vi "SEK2020v1SubVIIrParaOrigem00.vi"(8 "Parâmetros":T1={"Azul Max EV3 Cor"=17, "Azul Min EV3 Cor"=0, "Verde Max EV3 Cor"=6, "Verde Min EV3 Cor"=0, "Vermelho Max Ev3 Cor"=0, "Vermelho Min EV3 Cor"=0, "Chão EV3 Cor"=0.0, "Branco Max EV3 Cor"=0.0, "Branco Min EV3 Cor"=0.0, "Preto Max EV3 Cor"=0.0, "Preto Min EV3 Cor"=0.0, "Distância Tubulação"=0.0, "Distância Frontal"=0.0, "Amarelo Max EV3 Cor"=0.0, "Amarelo Min EV3 Cor"=0.0, "Distância Lateral"=0.0, "90°"=0.0, "180°"=0.0, "Seguidor de Linha"=0.0}, 11 "NXT/EV3":T2) -> (3 "NXT/EV3 2":T2)   [LabVIEW 2016]
uses:
  <vilib>/NXT/Subs/LVHSConnector.ctl
  <vilib>/NXT/LegoClasses/BrickReference/BrickReference.lvclass
  <vilib>/NXT/Block Support/NXT_OutputPort.ctl
  <vilib>/NXT/Block Support/NXT_InputPort.ctl
  <vilib>/NXT/Dual Mode Library/Sensors/EV3_Color_Reflect.vi
  <vilib>/NXT/NXTIO Xnodes/NXTIONodeSubVIs/NXTStopMotors.vi
  <vilib>/NXT/NXTIO Xnodes/AddressXNode/NXTIOAddress.xnode
  <vilib>/NXT/NXTIO Xnodes/NXTIOXNode/NXTIO.xnode
panel:
  out "x+1":i32
  in  "x":i32
  # "Sensor EV3 Cor"
  # "Sensor Ultrassônico"
  # "Sensor Giroscópio"
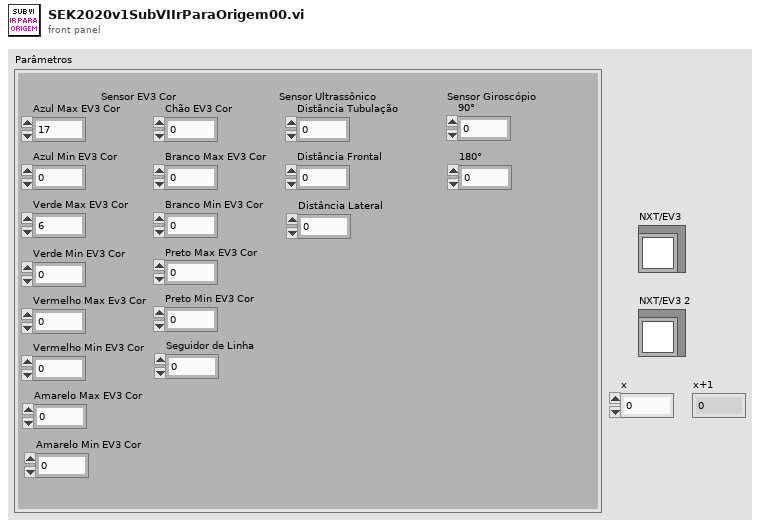
[diagram p1: front panel]
types:
  T1 = cluster{"Azul Max EV3 Cor":i32, "Azul Min EV3 Cor":i32, "Verde Max EV3 Cor":i32, "Verde Min EV3 Cor":i32, "Vermelho Max Ev3 Cor":i32, "Vermelho Min EV3 Cor":i32, "Chão EV3 Cor":sgl, "Branco Max EV3 Cor":sgl, "Branco Min EV3 Cor":sgl, "Preto Max EV3 Cor":sgl, "Preto Min EV3 Cor":sgl, "Distância Tubulação":sgl, "Distância Frontal":sgl, "Amarelo Max EV3 Cor":dbl, "Amarelo Min EV3 Cor":dbl, "Distância Lateral":sgl, "90°":sgl, "180°":sgl, "Seguidor de Linha":dbl}
  T2 = typedef "LVHSConnector.ctl" = refnum<class "BrickReference.lvclass">
  T3 = typedef "NXT_OutputPort.ctl" = u8
  T4 = typedef "NXT_InputPort.ctl" = u32
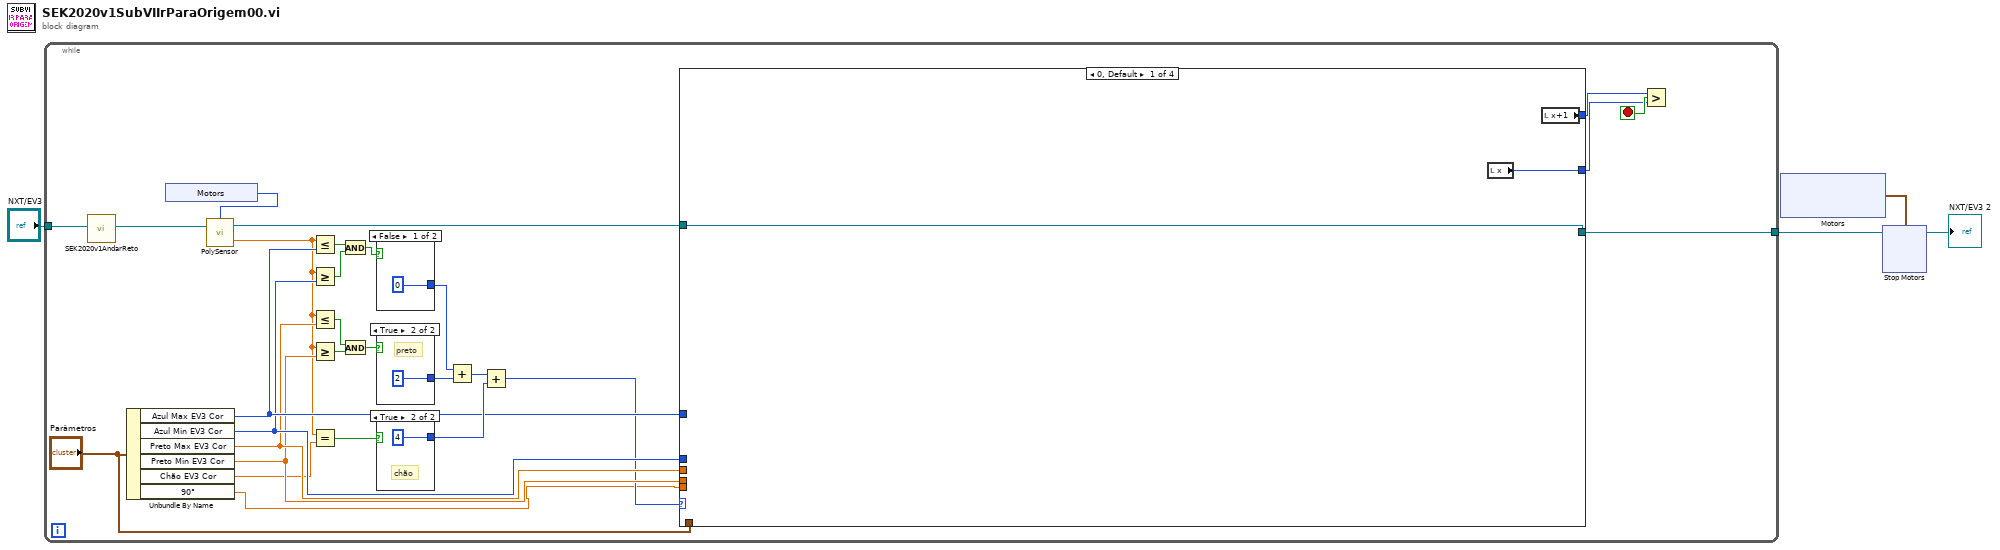
[diagram p0: block diagram]
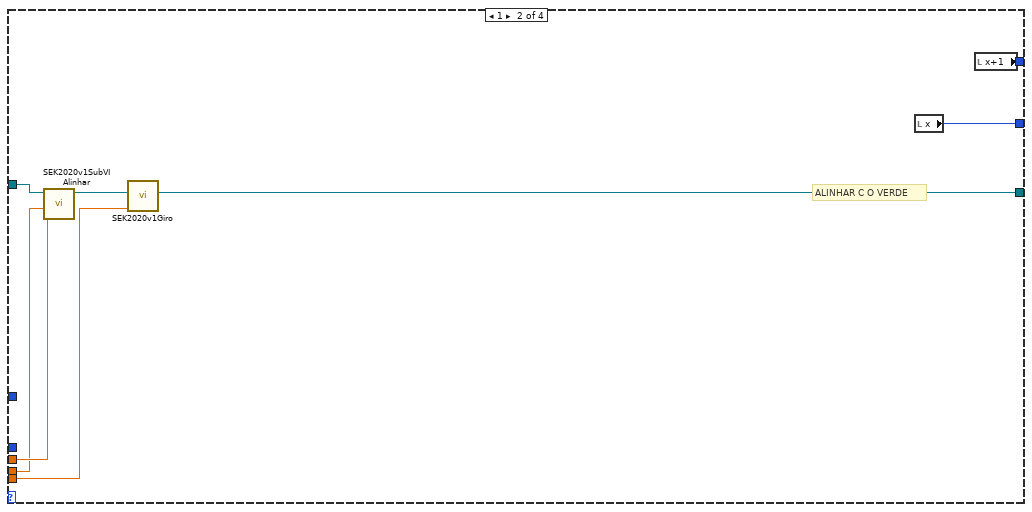
[diagram p2: hidden frame]
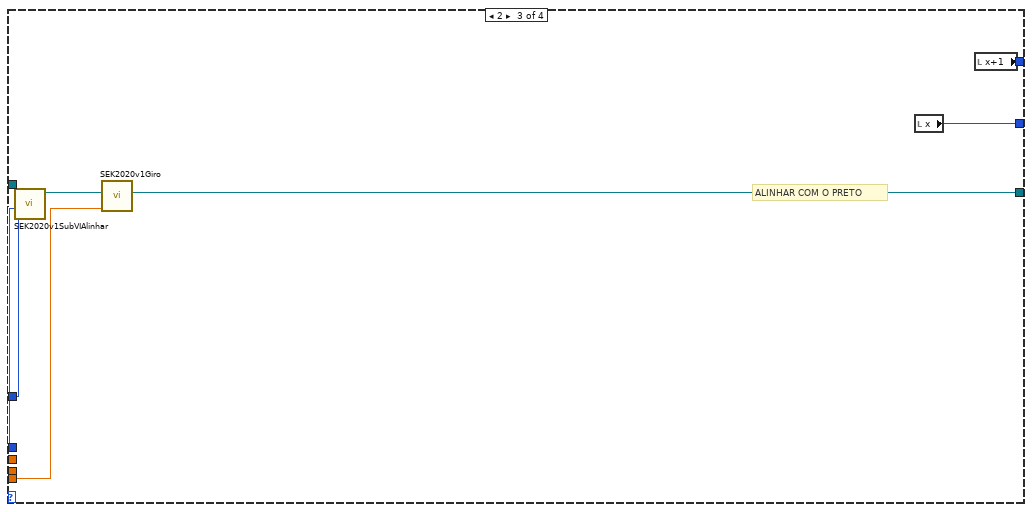
[diagram p3: hidden frame]
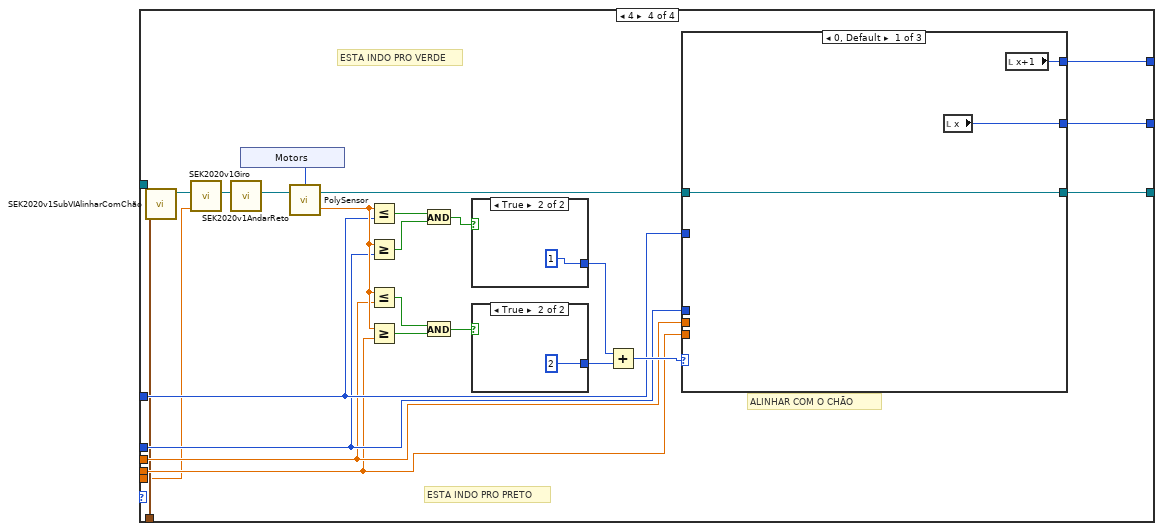
[diagram p4: hidden frame]
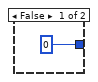
[diagram p5: hidden frame]
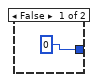
[diagram p6: hidden frame]
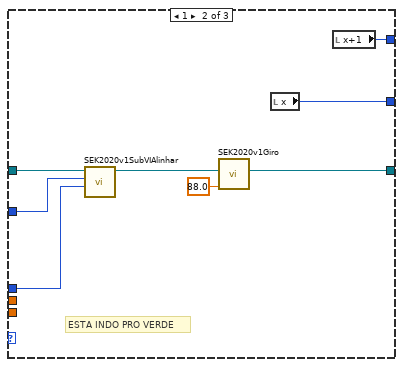
[diagram p7: hidden frame]
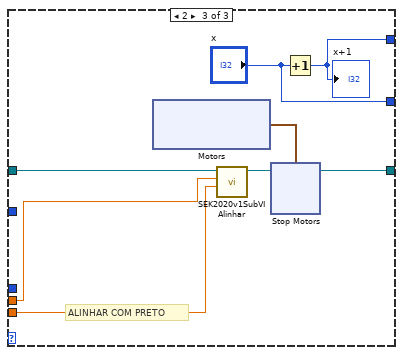
[diagram p8: hidden frame]
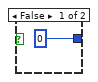
[diagram p9: hidden frame]
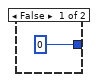
[diagram p10: hidden frame]
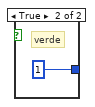
[diagram p11: hidden frame]
diagram:
  n1 = while {
    tunnel: "NXT/EV3" -> [w22]
    tunnel: [w7] -> w1
    stop <- w21 stop-if-true
    n2 = call "SEK2020v1AndarReto.vi"("NXT/EV3"=w22) -> ("NXT/EV3 2"=w10:T2)  [unwired: 9 in]
    n3 = Unbundle By Name("Parâmetros") -> ("Azul Max EV3 Cor"=w20:i32, "Azul Min EV3 Cor"=w19:i32, "Preto Max EV3 Cor"=w18:sgl, "Preto Min EV3 Cor"=w17:sgl, "Chão EV3 Cor"=w15:sgl, "90°"=w6:sgl)
    n4 = xnode "Motors"() -> ("Sensor"=w16:T4)
    n5 = call-poly <vilib>:"PolySensor.vi"("NXT/EV3"=w10, "Port (Port 1)"=w16) -> ("Scaled Value"=w12:sgl, "NXT/EV3"=w8:T2)  [unwired: 1 in]
    n6 = Less Or Equal?(x=w12, y=w20) -> (x <= y?=w25:bool)
    n7 = Greater Or Equal?(x=w12, y=w19) -> (x >= y?=w26:bool)
    n8 = Less Or Equal?(x=w12, y=w18) -> (x <= y?=w28:bool)
    n9 = Greater Or Equal?(x=w12, y=w17) -> (x >= y?=w27:bool)
    n10 = Equal?(x=w12, y=w15) -> (x = y?=w9:bool)
    n11 = And(x=w25, y=w26) -> (x .and. y?=w24:bool)
    n12 = And(x=w28, y=w27) -> (x .and. y?=w23:bool)
    n13 = case shown="False" w24 {
      tunnel: [0 1] -> w32
      frame False {
      }
      frame True {
        # "verde"
      }
    }
    n14 = case shown="True" w23 {
      tunnel: [0 2] -> w31
      frame False {
      }
      frame True {
        # "preto"
      }
    }
    n15 = case shown="True" w9 {
      tunnel: [0 4] -> w30
      frame False {
      }
      frame True {
        # "chão"
      }
    }
    n16 = Add(x=w32, y=w31) -> (x+y=w29:i32)
    n17 = Add(x=w29, y=w30) -> (x+y=w11:i32)
    n18 = case shown="0, Default" w11 {
      tunnel: w20 -> [_ _ w51 w65]
      tunnel: w19 -> [_ _ w52 w64]
      tunnel: w18 -> [_ w44 _ w63]
      tunnel: w17 -> [_ w43 _ w62]
      tunnel: w8 -> [w36 w42 w50 w77]
      tunnel: [w36 w38 w46 w60] -> w7
      tunnel: [w35 w40 w49 w59] -> w14
      tunnel: [w34 w41 w48 w58] -> w13
      tunnel: "Parâmetros" -> [_ _ _ w54]
      tunnel: w6 -> [_ w37 w45 w53]
      frame 0, Default {
        n19 = local read "x"() -> (w35:i32)
        n20 = local read "x+1"() -> (w34:i32)
      }
      frame 1 {
        # "ALINHAR C O VERDE"
        n21 = call "SEK2020v1SubVIAlinhar.vi"("Min EV3 Cor"=w43, "Max EV3 Cor"=w44, "NXT/EV3"=w42) -> ("NXT/EV3 2"=w39:T2)  [unwired: 8 in]
        n22 = call "SEK2020v1Giro.vi"("ANGULO"=w37, "NXT/EV3"=w39) -> ("NXT/EV3 2"=w38:T2)  [unwired: 6 in]
        n23 = local read "x"() -> (w40:i32)
        n24 = local read "x+1"() -> (w41:i32)
      }
      frame 2 {
        # "ALINHAR COM O PRETO"
        n25 = call "SEK2020v1SubVIAlinhar.vi"("Min EV3 Cor"=w52, "Max EV3 Cor"=w51, "NXT/EV3"=w50) -> ("NXT/EV3 2"=w47:T2)  [unwired: 8 in]
        n26 = call "SEK2020v1Giro.vi"("ANGULO"=w45, "NXT/EV3"=w47) -> ("NXT/EV3 2"=w46:T2)  [unwired: 6 in]
        n27 = local read "x"() -> (w49:i32)
        n28 = local read "x+1"() -> (w48:i32)
      }
      frame 4 {
        # "ESTA INDO PRO VERDE"
        # "ESTA INDO PRO PRETO"
        # "ALINHAR COM O CHÃO"
        n29 = call "SEK2020v1SubVIAlinharComChão.vi"("Parâmetros"=w54, "NXT/EV3"=w77) -> ("NXT/EV3 2"=w57:T2)  [unwired: 9 in]
        n30 = call "SEK2020v1Giro.vi"("ANGULO"=w53, "NXT/EV3"=w57) -> ("NXT/EV3 2"=w56:T2)  [unwired: 6 in]
        n31 = call "SEK2020v1AndarReto.vi"("NXT/EV3"=w56) -> ("NXT/EV3 2"=w71:T2)  [unwired: 9 in]
        n32 = xnode "Motors"() -> ("Sensor"=w55:T4)
        n33 = call-poly <vilib>:"PolySensor.vi"("NXT/EV3"=w71, "Port (Port 1)"=w55) -> ("Scaled Value"=w72:sgl, "NXT/EV3"=w61:T2)  [unwired: 1 in]
        n34 = Less Or Equal?(x=w72, y=w65) -> (x <= y?=w73:bool)
        n35 = Greater Or Equal?(x=w72, y=w64) -> (x >= y?=w74:bool)
        n36 = Less Or Equal?(x=w72, y=w63) -> (x <= y?=w76:bool)
        n37 = Greater Or Equal?(x=w72, y=w62) -> (x >= y?=w75:bool)
        n38 = And(x=w73, y=w74) -> (x .and. y?=w70:bool)
        n39 = And(x=w76, y=w75) -> (x .and. y?=w69:bool)
        n40 = case shown="True" w70 {
          tunnel: [0 1] -> w68
          frame False {
          }
          frame True {
          }
        }
        n41 = case shown="True" w69 {
          tunnel: [0 2] -> w67
          frame False {
          }
          frame True {
          }
        }
        n42 = Add(x=w68, y=w67) -> (x+y=w66:i32)
        n43 = case shown="0, Default" w66 {
          tunnel: w65 -> [_ w93 _]
          tunnel: w64 -> [_ w92 _]
          tunnel: w63 -> [_ _ w101]
          tunnel: w62 -> [_ _ w100]
          tunnel: w61 -> [w85 w91 w99]
          tunnel: [w85 w87 w94] -> w60
          tunnel: [w83 w89 w96] -> w58
          tunnel: [w84 w90 "x"] -> w59
          frame 0, Default {
            n44 = local read "x"() -> (w84:i32)
            n45 = local read "x+1"() -> (w83:i32)
          }
          frame 1 {
            # "ESTA INDO PRO VERDE"
            n46 = call "SEK2020v1SubVIAlinhar.vi"("Min EV3 Cor"=w92, "Max EV3 Cor"=w93, "NXT/EV3"=w91) -> ("NXT/EV3 2"=w88:T2)  [unwired: 8 in]
            n47 = call "SEK2020v1Giro.vi"("ANGULO"=sgl 88.0, "NXT/EV3"=w88) -> ("NXT/EV3 2"=w87:T2)  [unwired: 6 in]
            n48 = local read "x"() -> (w90:i32)
            n49 = local read "x+1"() -> (w89:i32)
          }
          frame 2 {
            # "ALINHAR COM PRETO"
            n50 = xnode "Motors"() -> ("Motor"=w98:cluster{"Port":T3, "Port":T3})
            n51 = call "SEK2020v1SubVIAlinhar.vi"("Min EV3 Cor"=w100, "Max EV3 Cor"=w101, "NXT/EV3"=w99) -> ("NXT/EV3 2"=w97:T2)  [unwired: 8 in]
            n52 = xnode "Stop Motors"("Motors"=w98, "NXT/EV3"=w97) -> ("NXT/EV3"=w94:T2)
            n53 = Increment(x="x") -> (x+1=w96:i32)
            "x+1" <- w96
          }
        }
      }
    }
    n54 = Greater?(x=w13, y=w14) -> (0:w21:bool)
  }
  n55 = xnode "Motors"() -> ("Motor"=w3:cluster{"Port":T3, "Port":T3})
  n56 = xnode "Stop Motors"("Motors"=w3, "NXT/EV3"=w1) -> ("NXT/EV3"=→"NXT/EV3 2":T2)
